vi "PMA Rohwerte FGV.vi"(0 "Messwerte":u16[](array[numeric]), 5 "Diagnose Werte":u16[](array[numeric]), 7 "Status":bool[](array[boolean]), 9 "Messbereich":u16[](array[numeric]), 13 "Aktion":T3) -> (4 "Messwerte":sgl[](array[numeric]) format="%#.3f", 6 "Diagnose Werte":T1, 8 "Status":T2, 10 "Messbereich":sgl[](array[numeric]) format="%#.3f")   [LabVIEW 2020, in "ABB-EL3000.lvlib" / "PMA.lvlib"]
uses:
  PMA.lvlib
  Aktion FGV Messwerte.ctl
  Allgemeine VI/Allgemeine VI.lvlib
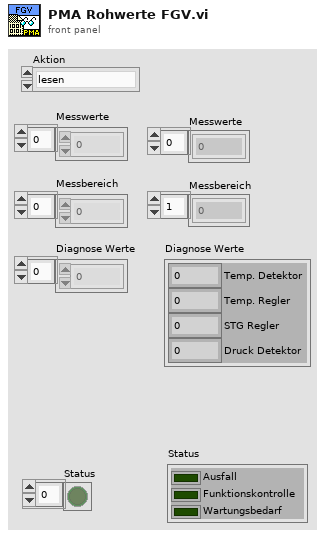
[diagram p1: front panel]
types:
  T1 = cluster{"Temp. Detektor":sgl, "Temp. Regler":sgl, "STG Regler":sgl, "Druck Detektor":sgl}
  T2 = cluster{"Ausfall":bool, "Funktionskontrolle":bool, "Wartungsbedarf":bool}
  T3 = typedef "ABB-EL3000.lvlib/PMA.lvlib/Aktion FGV Messwerte.ctl" = enum16{"lesen", "Messwerte", "Messbereich", "Status", "Diagnose Werte"}
  T4 = cluster{"Status[0]":bool, "Status[1]":bool, "Status[2]":bool}
  T5 = cluster{"Werte[0]":sgl, "Werte[1]":sgl, "Werte[2]":sgl, "Werte[3]":sgl}
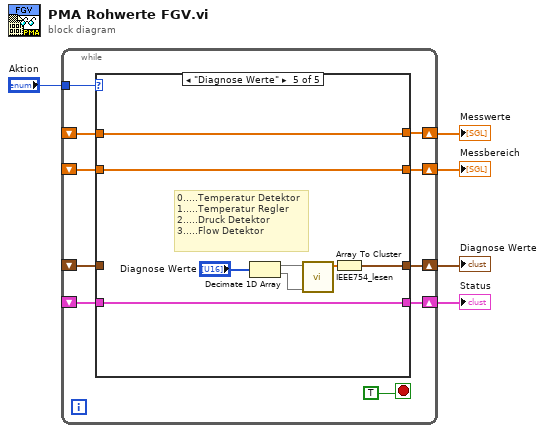
[diagram p0: block diagram]
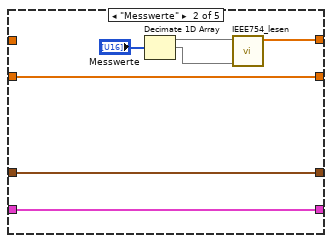
[diagram p3: hidden frame]
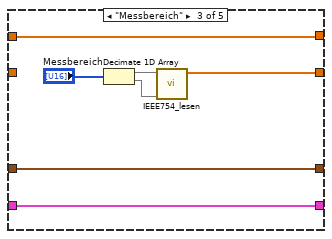
[diagram p4: hidden frame]
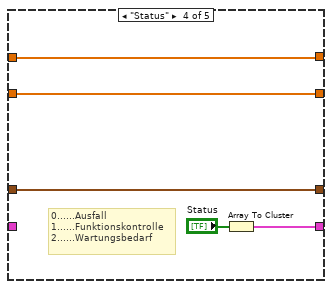
[diagram p5: hidden frame]
diagram:
  n1 = while {
    tunnel: "Aktion" -> [w14]
    shift-right: [w13] -> w4
    shift-left: _ -> [w12]
    shift-right: [w11] -> w3
    shift-left: _ -> [w10]
    shift-right: [w9] -> w2
    shift-left: _ -> [w8]
    shift-right: [w7] -> w1
    shift-left: _ -> [w6]
    stop <- TRUE stop-if-true
    n2 = case shown="\"Diagnose Werte\"" w14 {
      tunnel: [w19 w21 w33 w38 w46] -> w13
      tunnel: w12 -> [w19 _ w33 w38 w46]
      tunnel: [w18 w26 w32 w37 w45] -> w11
      tunnel: w10 -> [w18 w26 _ w37 w45]
      tunnel: [w17 w25 w31 w36 w39] -> w9
      tunnel: w8 -> [w17 w25 w31 w36 _]
      tunnel: [w16 w24 w30 w34 w44] -> w7
      tunnel: w6 -> [w16 w24 w30 _ w44]
      frame "lesen", Default {
      }
      frame "Messwerte" {
        n3 = Decimate 1D Array("Messwerte") -> (w22:u16[], w20:u16[])  [unwired: 1 out]
        n4 = call "IEEE754_lesen.vi"("lo"=w20, "hi"=w22) -> ("Werte"=w21:sgl[])  [unwired: 9 in]
      }
      frame "Messbereich" {
        n5 = Decimate 1D Array("Messbereich") -> (w28:u16[], w27:u16[])
        n6 = call "IEEE754_lesen.vi"("lo"=w27, "hi"=w28) -> ("Werte"=w32:sgl[])  [unwired: 9 in]
      }
      frame "Status" {
        # "0......Ausfall\n1......Funktionskontrolle\n2......Wartungsbedarf"
        n7 = Array To Cluster(array="Status") -> (cluster=w34:T4)
      }
      frame "Diagnose Werte" {
        # "0.....Temperatur Detektor\n1.....Temperatur Regler\n2.....Druck Detektor\n3.....Flow Detektor"
        n8 = Decimate 1D Array("Diagnose Werte") -> (w43:u16[], w42:u16[])
        n9 = call "IEEE754_lesen.vi"("lo"=w42, "hi"=w43) -> ("Werte"=w40:sgl[])  [unwired: 9 in]
        n10 = Array To Cluster(array=w40) -> (cluster=w39:T5)
      }
    }
  }
  "Messwerte" <- w4
  "Messbereich" <- w3
  "Status" <- w1
  "Diagnose Werte" <- w2
